vi "HeatCapacitor.vi"(7 "Capacity (J/K)":dbl, 11 "Transfer (J)":dbl) -> (2 "Temperature (K)":dbl, 3 "Heat (J)":dbl)   [LabVIEW 2023]
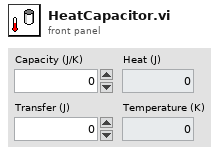
[diagram p1: front panel]
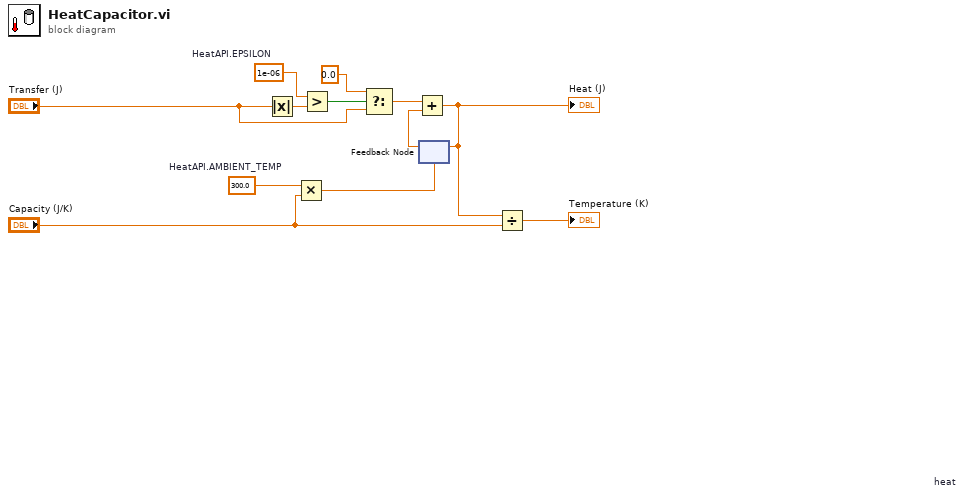
[diagram p0: block diagram]
diagram:
  w3 = 300.0  # HeatAPI.AMBIENT_TEMP
  w12 = 1e-06  # HeatAPI.EPSILON
  n1 = Absolute Value(x="Transfer (J)") -> (abs(x)=w11:dbl)
  n2 = Multiply(x=w3, y="Capacity (J/K)") -> (x*y=w2:dbl)
  n3 = Greater?(x=w12, y=w11) -> (0:w10:bool)
  n4 = Select(t=0.0, s=w10, f="Transfer (J)") -> (s? t:f=w9:dbl)
  n5 = feedback #1 "heat"(w2) -> (w8:dbl)
  n6 = Add(x=w9, y=w8) -> (x+y=w5:dbl)
  "Heat (J)" <- w5
  n7 = feedback-in #1(w5) -> ()
  n8 = Divide(x=w5, y="Capacity (J/K)") -> (x/y=→"Temperature (K)":dbl)
